vi "Process SCON_SPOS.vi"(11 "FHPP in":refnum<class "FHPP.lvclass">) -> (2 "Operation Mode":T1, 3 "FHPP out":refnum<class "FHPP.lvclass">)   [LabVIEW 2022 SP3, in "FHPP.lvclass"]
uses:
  FHPP.lvclass
  FHPP.lvclass/FHPP.ctl
  TypeDefs/Operating Mode.ctl
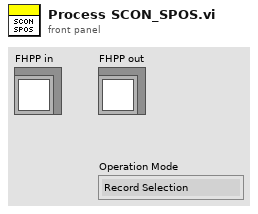
[diagram p1: front panel]
types:
  T1 = typedef "FHPP.lvclass/Operating Mode.ctl" = enum16{"Record Selection", "Direct Mode", "Reserved 1", "Reserved 2"}
  T2 = typedef "FHPP.lvclass/SPOS.ctl" = cluster{"Halt":bool, "Ack Start":bool, "Motion Complete":bool, "Ack Teach":bool, "Axis Moving":bool, "Drag Error":bool, "Standstill Control":bool, "Axis Referenced":bool}
  T3 = typedef "FHPP.lvclass/SCON.ctl" = cluster{"Drive Enabled":bool, "Operation Enabled":bool, "Warning":bool, "Error":bool, "Load Voltage Applied":bool, "FCT/MMI":bool, "Operation Mode":T1}
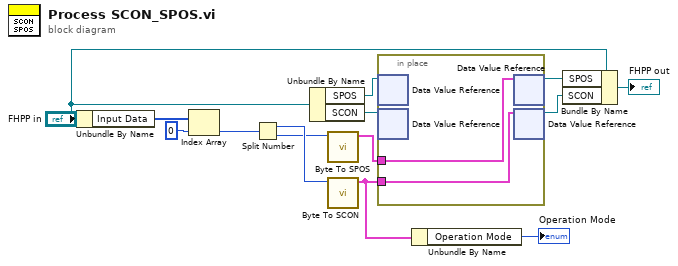
[diagram p0: block diagram]
diagram:
  n1 = Unbundle By Name("FHPP in") -> ("Input Data"=w7:u16[])
  n2 = Index Array(array=w7, index=0) -> (element=w4:u16)
  n3 = Split Number(x=w4) -> (hi(x)=w6:u8, lo(x)=w5:u8)
  n4 = Unbundle By Name("FHPP in") -> ("SPOS"=w9:refnum<data-value>, "SCON"=w10:refnum<data-value>)
  n5 = call "Byte To SPOS.vi"("Numeric"=w5) -> ("SPOS"=w11:T2)  [unwired: 10 in]
  n6 = call "Byte To SCON.vi"("Numeric"=w6) -> ("SCON"=w2:T3)  [unwired: 10 in]
  n7 = in-place {
    in-place-border: w2 -> [w16]
    in-place-border: w11 -> [w15]
    n8 = in-place-dvr #1(w9) -> ()  [unwired: 2 out]
    n9 = in-place-dvr #2(w10) -> ()  [unwired: 2 out]
    n10 = in-place-dvr #1(w15) -> (w13:refnum<data-value>)  [unwired: 1 out]
    n11 = in-place-dvr #2(w16) -> (w14:refnum<data-value>)  [unwired: 1 out]
  }
  n12 = Unbundle By Name(w2) -> ("Operation Mode"=→"Operation Mode":T1)
  n13 = Bundle By Name(cluster="FHPP in", "SPOS"=w13, "SCON"=w14) -> (→"FHPP out":refnum<class "FHPP.lvclass">)
